vi "Helper SubVI - Filters Selection.vi"(8 "error in (no error)":errorcluster, 10 "wavelet":u16(ring) items=["db02"=0, "db03"=1, "db04"=2, "db05"=3, "db06"=4, "db07"=5, "db08"=6, "db09"=7, "db10"=8, "db11"=9, "db12"=10, "db13"=11, "db14"=12, "Haar"=13, "bior1_3"=14, "bior1_5"=15, "bior2_2"=16, "bior2_4"=17, "bior2_6"=18, "bior2_8"=19, "bior3_1"=20, "bior3_3"=21, "bior3_5"=22, "bior3_7"=23, "bior3_9"=24, "bior4_4 (FBI)"=25, "bior5_5"=38, "bior6_8"=39, "coif1"=26, "coif2"=27, "coif3"=28, "coif4"=29, "coif5"=30, "sym2"=31, "sym3"=32, "sym4"=33, "sym5"=34, "sym6"=35, "sym7"=36, "sym8"=37], 11 "filters":cluster{"lowpass":dbl[], "highpass":dbl[]}) -> (0 "error out":errorcluster, 2 "synthesis filters":cluster{"lowpass":dbl[], "highpass":dbl[]}, 3 "analysis filters":cluster{"lowpass":dbl[], "highpass":dbl[]})   [LabVIEW 2023]
doc: "Selects the analysis filters and the synthesis filters."
uses:
  <vilib>/addons/_Advanced Signal Processing/NI_AdvSigProcWA.lvlib
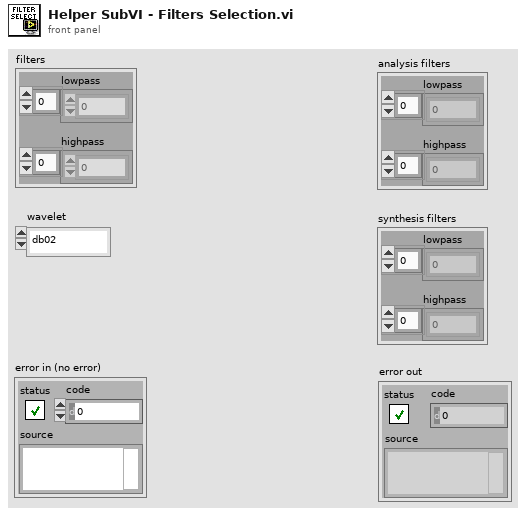
[diagram p1: front panel]
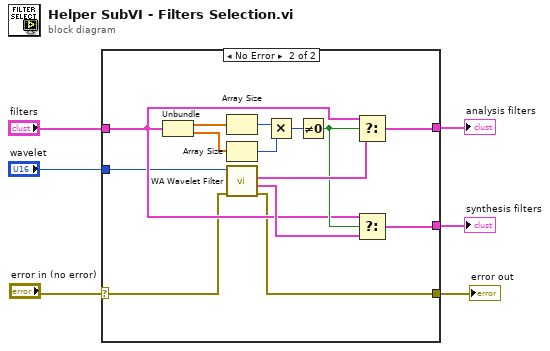
[diagram p0: block diagram]
diagram:
  n1 = case shown="No Error" "error in (no error)" {
    selector: "error in (no error)" -> [w7 w9]
    tunnel: [_ w20] -> w6
    tunnel: "filters" -> [_ w12]
    tunnel: [_ w11] -> w4
    tunnel: "wavelet" -> [_ w10]
    tunnel: [w7 w8] -> w1
    frame Error {
    }
    frame No Error {
      n2 = Unbundle(w12) -> ("lowpass"=w15:dbl[], "highpass"=w16:dbl[])
      n3 = Array Size(array=w15) -> (size(s)=w18:i32)
      n4 = Array Size(array=w16) -> (size(s)=w17:i32)
      n5 = call <vilib>:"WA Wavelet Filter.vi"("error in (no error)"=w9, "wavelet"=w10) -> ("error out"=w8:errorcluster, "synthesis filters"=w13:cluster{"lowpass":dbl[], "highpass":dbl[]}, "analysis filters"=w21:cluster{"lowpass":dbl[], "highpass":dbl[]})  [unwired: 2 in, 5 out]
      n6 = Multiply(x=w18, y=w17) -> (x*y=w19:i32)
      n7 = Not Equal To 0?(x=w19) -> (x != 0?=w14:bool)
      n8 = Select(t=w12, s=w14, f=w21) -> (s? t:f=w20:cluster{"lowpass":dbl[], "highpass":dbl[]})
      n9 = Select(t=w12, s=w14, f=w13) -> (s? t:f=w11:cluster{"lowpass":dbl[], "highpass":dbl[]})
    }
  }
  "analysis filters" <- w6
  "synthesis filters" <- w4
  "error out" <- w1
